vi "ATF Storage-Data transfer_C.vi"(2 "Message Queue":refnum<queue>, 3 "error constant":errorcluster) -> (10 "error out":errorcluster)   [LabVIEW 2022 SP3]
uses:
  <vilib>/Platform/TimedLoop/XDataNode/wakeup.ctl
  <vilib>/Platform/TimedLoop/XDataNode/XDNodeRunTimeDep.lvlib
  <vilib>/Platform/TimedLoop/XDataNode/nitl_modes.ctl
  <vilib>/Platform/TimedLoop/XDataNode/timing_clust.ctl
  <vilib>/platform/TimedLoop/XDataNode/XDataNode.xnode
  <resource>/objmgr/ni.dex.rc
  <vilib>/ErrorRing/Error Ring.xnode
  Pumb PXie/RT Support/ATF-Pump-RT_Global_R.vi
  RT Controls/ATF Storage-Data Type Control screen.ctl
panel:
  out "Write Backlog":i32
  out "Loop Delay":u32
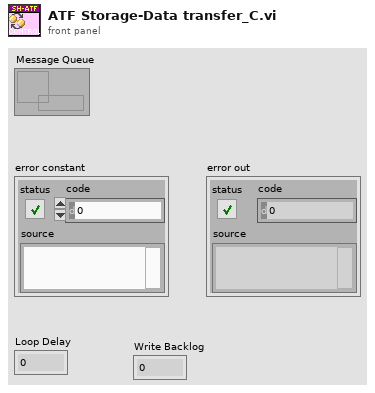
[diagram p1: front panel]
types:
  T1 = typedef "ATF Storage-Data Type Control screen.ctl" = cluster{"DI_Data":digitalwaveform[], "Drive_A_C":waveform(dbl)[], "Drive_A_D":waveform(dbl)[], "Drive_L_C":waveform(dbl)[], "Drive_L_D":waveform(dbl)[], "Loop Status":bool[], "CDT Timer":dbl, "RT Error":cluster{"Error Code":string, "Error Source":string}, "DO":waveform(dbl)[], "SEQ Monitor":string[], "Device List":string}
  T2 = enum16{"Init", "Read 'All'", "Read 'n'", "Read '1'", "Write '1'", "Write 'n'", "Write 'All'"}
  T3 = typedef "XDNodeRunTimeDep.lvlib/timing_clust.ctl" = cluster{"Expected End [f-1]":u64, "Actual End [f-1]":u64, "Finished Late? [f-1]":bool, "Expected End [i-1]":u64, "Actual End [i-1]":u64, "Finished Late? [i-1]":bool, "Expected Start [i]":u64, "Actual Start [i]":u64, "Expected Start [f]":u64, "Actual Start [f]":u64, "Source Name":string, "Structure Name":string, "Period":i64, "Deadline":i64, "Offset":i64, "Start":i64, "Priority":i32, "Timeout":i32, "Mode":T4, "Wakeup Reason":T5, "Error":errorcluster, "Source Type":string, "Secondary Source Type":string, "Global End Time":u64, "Global Start Time":u64, "Frame Duration":u64, "Iteration Duration":u64, "Assigned CPU":i32, "I/O Scan Engine Mode":u32}
  T4 = typedef "XDNodeRunTimeDep.lvlib/nitl_modes.ctl" = enum32{"No Change", "Process missed periods, maintain original phase", "Discard missed periods, maintain original phase", "Process missed periods, ignore original phase", "Discard missed periods, ignore original phase"}
  T5 = typedef "XDNodeRunTimeDep.lvlib/wakeup.ctl" = enum32{"Normal", "Aborted", "Asynchronous wakeup", "Timing source error", "Timed loop error", "Timeout"}
  T6 = cluster{"Error Code":string, "Error Source":string}
  T7 = cluster{"Start DAQ":bool, "Stop DAQ":bool, "RT Stop":bool, "RT Exit":bool, "Start Seq":bool}
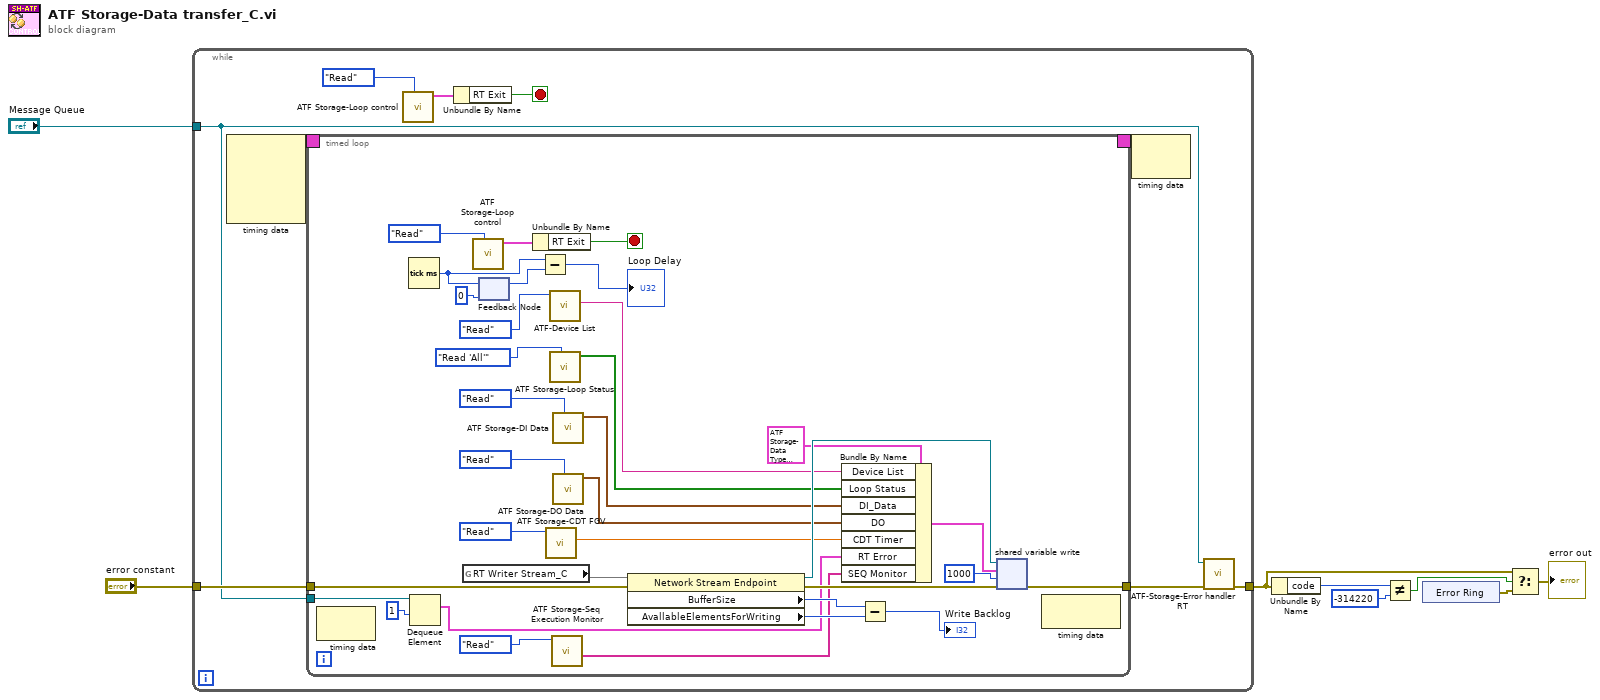
[diagram p0: block diagram]
diagram:
  n1 = while {
    tunnel: "error constant" -> [w17]
    tunnel: [w12] -> w3
    tunnel: "Message Queue" -> [w11]
    stop <- w14 stop-if-true
    n2 = node-c288() -> (w10:T3)  [unwired: 4 in]
    n3 = timed-loop {
      tunnel: w17 -> [w44]
      tunnel: [w43] -> w13
      timing: w10 -> [_]
      timing-out: [_] -> w9
      tunnel: w11 -> [w29]
      stop <- w35 stop-if-true
      n4 = node-c288() -> ()  [unwired: 1 in, 1 out]
      n5 = Tick Count (ms)() -> (millisecond timer value=w40:u32)
      n6 = Dequeue Element(queue=w29, timeout in ms (-1)=1) -> (element=w26:T6)  [unwired: 1 in, 3 out]
      n7 = global read "ATF-Pump-RT_Global_R.vi" "RT Writer Stream_C"() -> (w38)
      n8 = call "ATF Storage-Loop control.vi"("Action"=enum16{"Init", "Write", "Read"}."Read") -> ("Loop Control out"=w37:T7)  [unwired: 9 in, 1 out]
      n9 = feedback #1(u32 0 ("millisecond timer value")) -> (w41:u32)
      n10 = feedback-in #1(w40) -> ()
      n11 = Unbundle By Name(w37) -> ("RT Exit"=w35:bool)
      n12 = Subtract(x=w40, y=w41) -> (x-y=→"Loop Delay":u32)
      n13 = call "ATF Storage-CDT FGV.vi"("Write/Read"=enum16{"Write", "Read"}."Read") -> ("CDT Out"=w27:dbl)  [unwired: 9 in, 1 out]
      n14 = call "ATF-Device List.vi"("Enum"=enum16{"Write", "Read"}."Read") -> ("DL 2"=w18:string)  [unwired: 9 in, 1 out]
      n15 = call "ATF Storage-Loop Status.vi"("Option"=T2."Read 'All'") -> ("Status List Out"=w33:bool[])  [unwired: 8 in, 2 out]
      n16 = call "ATF Storage-Seq Execution Monitor.vi"("Enum"=enum16{"Read", "Write "}."Read") -> ("Seq Monitor"=w24:string[])  [unwired: 9 in, 1 out]
      n17 = call "ATF Storage-DI Data.vi"("Enum"=enum16{"Write", "Read"}."Read") -> ("Out_DI data"=w22:digitalwaveform[])  [unwired: 10 in]
      n18 = call "ATF Storage-DO Data.vi"("Enum"=enum16{"Write", "Read"}."Read") -> ("out_DO data"=w20:waveform(dbl)[])  [unwired: 10 in]
      n19 = property class="Network Stream Endpoint"(reference=w38, error in=w44) -> (reference out=w49:refnum<k21>, error out=w45:errorcluster, "BufferSize"=w48:i32, "AvallableElementsForWriting"=w47:i32)
      n20 = Bundle By Name(cluster=T1 {"DI_Data"=[], "Drive_A_C"=[], "Drive_A_D"=[], "Drive_L_C"=[], "Drive_L_D"=[], "Loop Status"=[], "CDT Timer"=0.0, "RT Error"={"Error Code"="", "Error Source"=""}, "DO"=[], "SEQ Monitor"=[], "Device List"=""} ("Cluster"), "Device List"=w18, "Loop Status"=w33, "DI_Data"=w22, "DO"=w20, "CDT Timer"=w27, "RT Error"=w26, "SEQ Monitor"=w24) -> (w31:T1)
      n21 = Subtract(x=w48, y=w47) -> (x-y=→"Write Backlog":i32)
      n22 = shared-variable-write(w49, w45, w31, 1000 ("timeout ms (-1)")) -> (w43:errorcluster)  [unwired: 2 out]
      n23 = node-c288() -> ()  [unwired: 1 in, 1 out]
    }
    n24 = call "ATF Storage-Loop control.vi"("Action"=enum16{"Init", "Write", "Read"}."Read") -> ("Loop Control out"=w16:T7)  [unwired: 9 in, 1 out]
    n25 = Unbundle By Name(w16) -> ("RT Exit"=w14:bool)
    n26 = node-c288(w9) -> ()  [unwired: 1 out]
    n27 = call "ATF-Storage-Error handler RT.vi"("error in"=w13, "Message Queue"=w11) -> ("error out"=w12:errorcluster)  [unwired: 8 in, 1 out]
  }
  n28 = Unbundle By Name(w3) -> ("code"=w8:i32)
  n29 = Not Equal?(x=w8, y=-314220) -> (x != y?=w5:bool)
  n30 = xnode "Error Ring"() -> ("error out"=w4:errorcluster)
  n31 = Select(t=w3, s=w5, f=w4) -> (s? t:f=→"error out":errorcluster)
